vi "GetInputPadsList.vi"(10 "Input Index":i32, 11 "Pads Array":T1(array[cluster])) -> (3 "Input Pads List":u32[](array[numeric]))   [LabVIEW 2012, in "Virtual-PGA.lvlib"]
uses:
  Virtual-PGA.lvlib
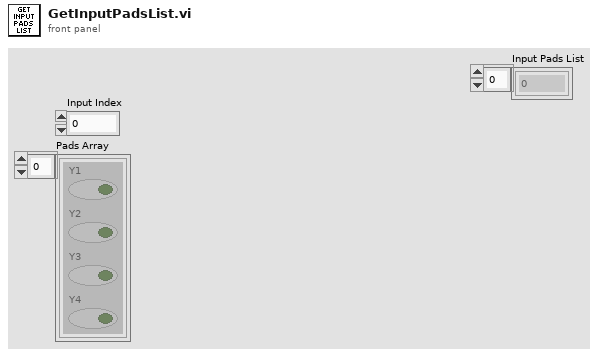
[diagram p1: front panel]
types:
  T1 = cluster{"Y1":bool, "Y2":bool, "Y3":bool, "Y4":bool}[]
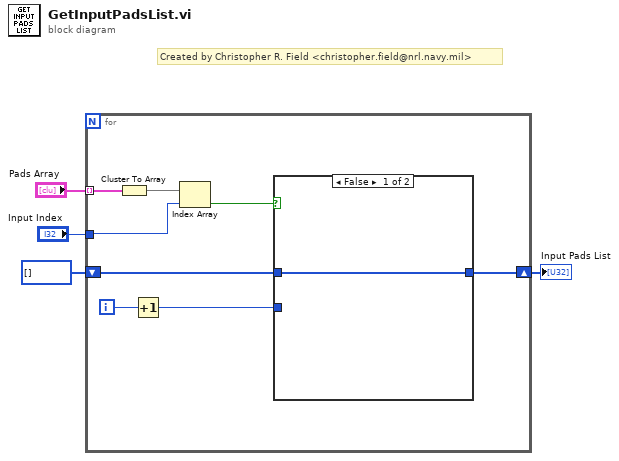
[diagram p0: block diagram]
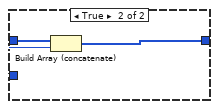
[diagram p2: hidden frame]
diagram:
  # "Created by Christopher R. Field <christopher.field@nrl.navy.mil>"
  n1 = for {
    tunnel: "Pads Array" -> [w8] mode=indexing
    shift-right: [w9] -> w1
    shift-left: u32[] [] -> [w12]
    tunnel: "Input Index" -> [w5]
    i -> [w11]
    n2 = Cluster To Array(cluster=w8) -> (array=w7:bool[])
    n3 = Increment(x=w11) -> (x+1=w10:i32)
    n4 = Index Array(array=w7, index=w5) -> (element=w6:bool)
    n5 = case shown="False" w6 {
      tunnel: w12 -> [w13 w16]
      tunnel: w10 -> [_ w15]
      tunnel: [w13 w14] -> w9
      frame False {
      }
      frame True {
        n6 = Build Array (concatenate)(w16, w15) -> (w14:u32[])
      }
    }
  }
  "Input Pads List" <- w1
